vi "RunErrorCode.vi"(10 "previous #":i32, 11 "previous time":timestamp) -> (1 "Run":bool, 2 "Number of Error Files":i32, 3 "current time":timestamp)   [LabVIEW 2012]
panel:
  out "New File?":bool
  out "last mod":timestamp
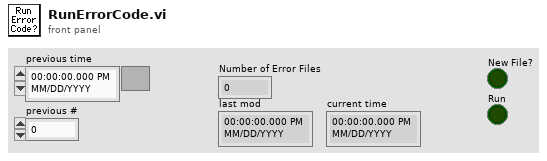
[diagram p1: front panel]
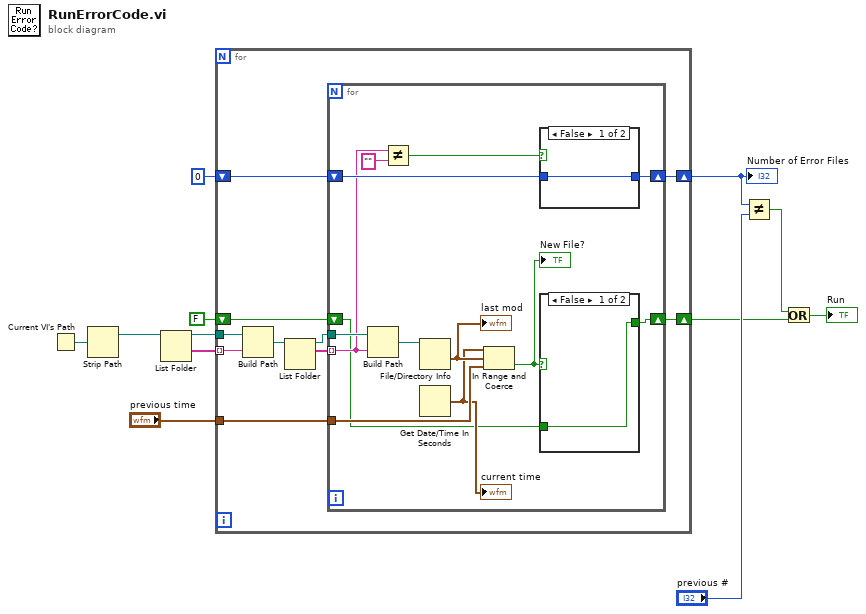
[diagram p0: block diagram]
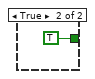
[diagram p2: hidden frame]
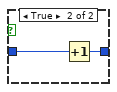
[diagram p3: hidden frame]
diagram:
  n1 = Current VI's Path() -> (path=w12:path)
  n2 = Strip Path(path=w12) -> (stripped path=w11:path)  [unwired: 1 out]
  n3 = List Folder(path=w11) -> (path out=w10:path, folder names=w9:string[])  [unwired: 3 in, 2 out]
  n4 = for {
    tunnel: w10 -> [w21]
    tunnel: w9 -> [w20] mode=indexing
    shift-right: [w16] -> w6
    shift-left: 0 -> [w17]
    tunnel: "previous time" -> [w15]
    shift-right: [w14] -> w2
    shift-left: FALSE -> [w13]
    n5 = Build Path(base path=w21, name or relative path=w20) -> (appended path=w22:path)
    n6 = List Folder(path=w22) -> (path out=w19:path, filenames=w18:string[])  [unwired: 3 in, 2 out]
    n7 = for {
      tunnel: w19 -> [w30]
      tunnel: w18 -> [w29] mode=indexing
      shift-right: [w32] -> w16
      shift-left: w17 -> [w33]
      tunnel: w15 -> [w28]
      shift-right: [w24] -> w14
      shift-left: w13 -> [w23]
      n8 = Build Path(base path=w30, name or relative path=w29) -> (appended path=w31:path)
      n9 = Not Equal?(x=w29, y="") -> (x != y?=w35:bool)
      n10 = File/Directory Info(path=w31) -> (last mod=w27:timestamp)  [unwired: 1 in, 6 out]
      "last mod" <- w27
      n11 = Get Date/Time In Seconds() -> (seconds since 1Jan1904=w26:timestamp)
      "current time" <- w26
      n12 = In Range and Coerce(upper limit=w26, x=w27, lower limit=w28) -> (In Range?=w25:bool)  [unwired: 1 out]
      "New File?" <- w25
      n13 = case shown="False" w35 {
        tunnel: w33 -> [w38 w40]
        tunnel: [w38 w39] -> w32
        frame False {
        }
        frame True {
          n14 = Increment(x=w40) -> (x+1=w39:i32)
        }
      }
      n15 = case shown="False" w25 {
        tunnel: [w36 TRUE] -> w24
        tunnel: w23 -> [w36 _]
        frame False {
        }
        frame True {
        }
      }
    }
  }
  "Number of Error Files" <- w6
  n16 = Not Equal?(x=w6, y="previous #") -> (x != y?=w4:bool)
  n17 = Or(x=w4, y=w2) -> (x .or. y?=→"Run":bool)
